vi "Open (HTTP).vi"(7 "configuration":refnum<class "NI Skyline Configuration HTTP.lvclass"> caption="configuration (system default)", 8 "error in (no error)":errorcluster) -> (0 "error out":errorcluster, 3 "message session":refnum<class "NI Skyline Message HTTP.lvclass">)   [LabVIEW 2020, in "NI Skyline Message HTTP.lvclass"]
doc: "Creates an HTTP message session with the server based on the SystemLink configuration information."
uses:
  NI Skyline Message HTTP.lvclass
  Configuration/Configuration HTTP_class/NI Skyline Configuration HTTP.lvclass
  Configuration/Configuration HTTP_class/NI Skyline Configuration HTTP.lvclass/NI Skyline Configuration HTTP.ctl
  NI Skyline Message HTTP.lvclass/NI Skyline Message HTTP.ctl
  HTTP/NI Skyline Message HTTP Library.lvlib
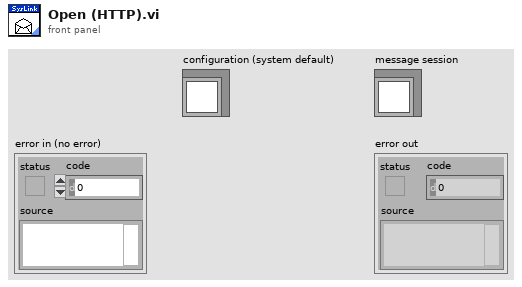
[diagram p1: front panel]
types:
  T1 = typedef "NI Skyline Configuration Library.lvlib/Configuration.ctl" = cluster{"Server URL":string, "Session":T2, "Raw Session Queue":refnum<queue>}
  T2 = typedef "LabVIEWHTTPClient.lvlib/ClientHandle.ctl" = refnum<k1>
  T3 = typedef "NI Skyline Message HTTP Library.lvlib/Message Session.ctl" = cluster{"Configuration":T1, "token":string}
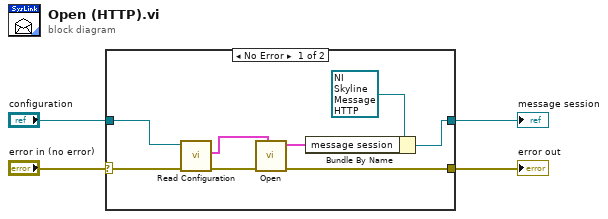
[diagram p0: block diagram]
diagram:
  n1 = case shown="No Error" "error in (no error)" {
    selector: "error in (no error)" -> [w7 w13]
    tunnel: [w10 _] -> w1
    tunnel: [w12 w13] -> w4
    tunnel: "configuration" -> [w6 _]
    frame No Error {
      n2 = call "Read Configuration.vi"("error in (no error)"=w7, "HTTP configuration in"=w6) -> ("error out"=w8:errorcluster, "configuration"=w5:T1)  [unwired: 7 in, 1 out]
      n3 = call "Open.vi"("configuration"=w5, "error in (no error)"=w8) -> ("error out"=w12:errorcluster, "message session"=w9:T3)  [unwired: 8 in]
      n4 = Bundle By Name(cluster=refnum<class "NI Skyline Message HTTP.lvclass"> refnum ("NI Skyline Message HTTP.lvclass 2"), "message session"=w9) -> (w10:refnum<class "NI Skyline Message HTTP.lvclass">)
    }
    frame Error {
    }
  }
  "error out" <- w4
  "message session" <- w1
